vi "stream_only_production.vi"() -> ()   [LabVIEW 2025, in "LabJackEKG.lvlib"]
uses:
  LabJackEKG.lvlib
  StreamProducerLoopData.ctl
panel:
  out "Numeric":i32
  out "Direction":i64
  out "error out 2":errorcluster
  out "FLOW":T1(graph)={"Flow [L/min]"=nan, "Flow [L/min]"=nan, "Flow [L/min]"=nan}
  out "stop":bool
  in  "RMS Sampling Window [s]":dbl
  in  "TC Sampling Window [s]":dbl=0.25
  in  "error in (no error)":errorcluster
  in  "TC Offset [V]":dbl[](array[numeric])=[0.0, 0.0]
  in  "TC Scale":dbl[](array[numeric])=[1.0, 1.0]
  in  "Flow L/pulse":dbl[](array[numeric])=[1.0, 1.0, 1.0]
  in  "Flow Min. Sampling Window [s]":dbl
  in  "Flow Max. Samping Window [s]":dbl
  out "TC [degC]":dbl[](array[numeric])
  out "RMS [V]":dbl[](array[numeric])=[nan, nan, nan, nan, nan, nan]
  in  "Drum Max. Samping Window [s]":dbl=1.0
  in  "Drum Min. Sampling Window [s]":dbl=0.25
  in  "Sampling Frequency [Hz]":dbl=250.0
  in  "ms":u32=100
  out "Waveform Chart":dbl(graph)=nan
  in  "Drum Reflectors":i64=4
  out "error out":errorcluster={"status"=TRUE, "code"=8607, "source"="LJM_eStreamStart.vi"}
  in  "stop":bool
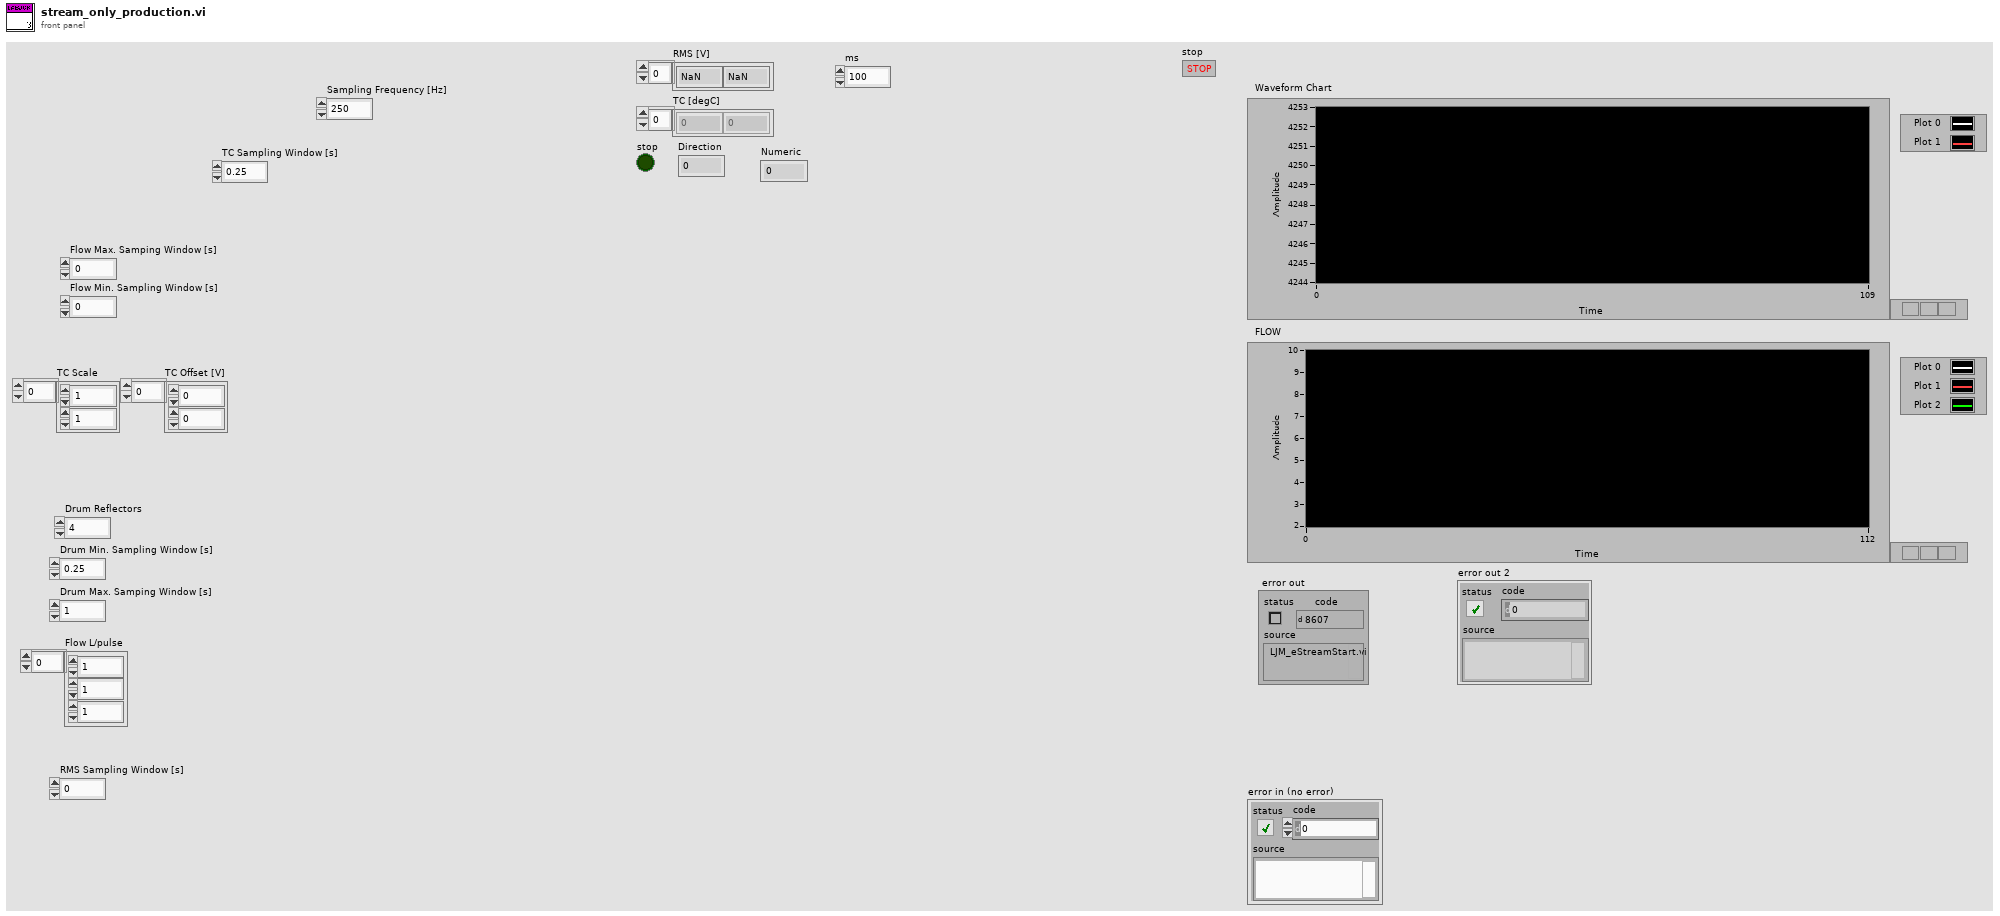
[diagram p1: front panel]
types:
  T1 = cluster{"Flow [L/min]":dbl, "Flow [L/min]":dbl, "Flow [L/min]":dbl}
  T2 = typedef "StreamProducerLoopData.ctl" = cluster{"Count":i64, "Time":i64, "Initialized":bool}
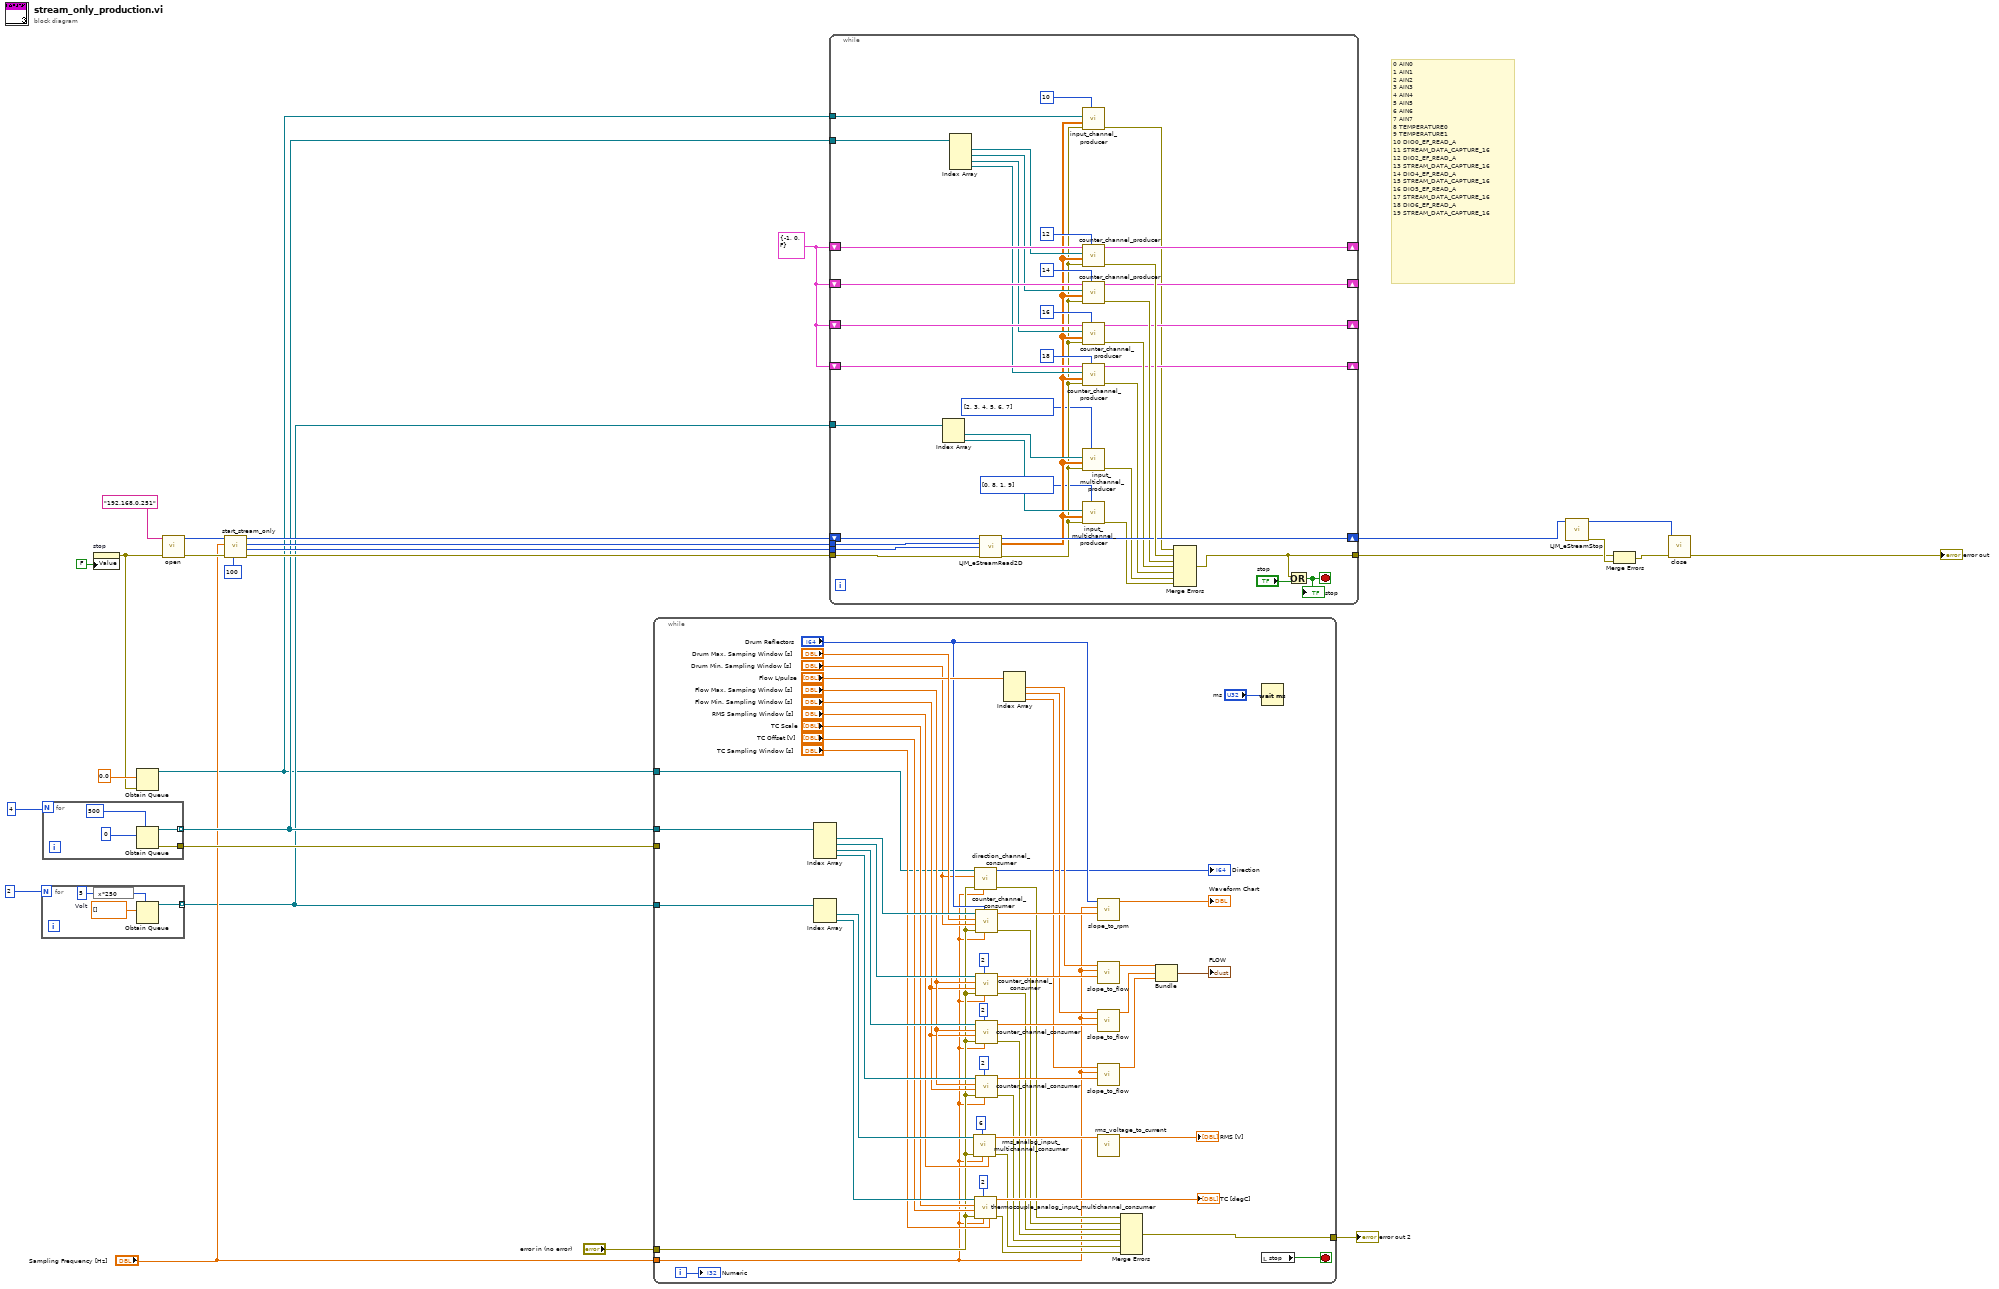
[diagram p0: block diagram]
diagram:
  w5 = T2 {"Count"=-1, "Time"=0, "Initialized"=FALSE} ("output cluster")
  # "0 AIN0\n1 AIN1\n2 AIN2\n3 AIN3\n4 AIN4\n5 AIN5\n6 AIN6\n7 AIN7\n8 TEMPERATURE0\n9 TEMPERATURE1\n10 DIO0_EF_READ_A\n11 STREAM_DATA_CAPTURE_16\n12 DIO2_EF_READ_A\n13 STREAM_DATA_CAPTURE_16\n14 DIO4_EF_READ_A\n15 STREAM_DATA_CAPTURE_16\n16 DIO5_EF_READ_A\n17 STREAM_DATA_CAPTURE_16\n18 DIO6_EF_READ_A\n19 STREAM_DATA_CAPTURE_16"
  n1 = for {
    N: 2 -> [_]
    tunnel: [w30] -> w8 mode=indexing
    w31 = dbl[] []  # Volt
    n2 = expression code="x*250"(5 ("max queue size (-1, unlimited)")) -> (w28:i32)
    n3 = Obtain Queue(max queue size (-1, unlimited)=w28, element data type=w31) -> (queue out=w30:refnum<queue>)  [unwired: 3 in, 2 out]
  }
  n4 = for {
    N: 4 -> [_]
    tunnel: [w35] -> w18
    tunnel: [w33] -> w17 mode=indexing
    n5 = Obtain Queue(max queue size (-1, unlimited)=500, element data type=i64 0) -> (queue out=w33:refnum<queue>, error out=w35:errorcluster)  [unwired: 3 in, 1 out]
  }
  n6 = property on="stop" class="Bool (strict)"("Value"=FALSE ("stop")) -> (error out=w1:errorcluster)  [unwired: 2 in, 1 out]
  n7 = Obtain Queue(element data type=0.0, error in (no error)=w1) -> (queue out=w3:refnum<queue>)  [unwired: 3 in, 2 out]
  n8 = call "open.vi"("error in"=w1, "IP Address (LJM_idANY )"="192.168.0.251") -> ("error out"=w27:errorcluster, "Handle"=w26:i32)  [unwired: 7 in, 1 out]
  n9 = call "start_stream_only.vi"("Period [ms]"=100, "error in (no error)"=w27, "Scan Rate (Hz)"="Sampling Frequency [Hz]", "Handle In"=w26) -> ("error out"=w25:errorcluster, "NumReadAddresses"=w22:i32, "ScansPerRead Out"=w23:i32, "Handle Out"=w24:i32)  [unwired: 4 in]
  n10 = while {
    tunnel: w17 -> [w83]
    tunnel: w18 -> [_]
    tunnel: "Sampling Frequency [Hz]" -> [w37]
    tunnel: w8 -> [w72]
    tunnel: "error in (no error)" -> [w40]
    tunnel: [w43] -> w6
    tunnel: w3 -> [w42]
    i -> [w36]
    stop <- w54 stop-if-true
    n11 = Index Array(array=w83) -> (element #1=w82:refnum<queue>, element #2=w81:refnum<queue>, element #3=w80:refnum<queue>, element #4=w79:refnum<queue>)  [unwired: 4 in]
    n12 = Index Array(array=w72) -> (element #1=w70:refnum<queue>, element #2=w71:refnum<queue>)  [unwired: 2 in]
    n13 = call "rms_analog_input_multichannel_consumer.vi"("Sampling Window [s]"="RMS Sampling Window [s]", "Sampling Frequency [Hz]"=w37, "Number of Channels"=6, "error in (no error)"=w40, "queue out"=w70) -> ("error out"=w48:errorcluster, "RMS [V]"=w69:dbl[])  [unwired: 5 in]
    n14 = call "direction_channel_consumer.vi"("Sampling Frequency [Hz]"=w37, "error in (no error)"=w40, "Sampling Offset [s]"="Drum Min. Sampling Window [s]", "Q"=w42) -> ("error out"=w39:errorcluster, "Direction"=→"Direction":i64)  [unwired: 6 in]
    n15 = call "thermocouple_analog_input_multichannel_consumer.vi"("Sampling Window [s]"="TC Sampling Window [s]", "Sampling Frequency [Hz]"=w37, "Number of Channels"=2, "error in (no error)"=w40, "Offset"="TC Offset [V]", "Scale"="TC Scale", "queue out"=w71) -> ("error out"=w49:errorcluster, "TC [degC]"=→"TC [degC]":dbl[])  [unwired: 1 in, 2 out]
    n16 = call "counter_channel_consumer.vi"("Sampling Frequency [Hz]"=w37, "Sample Group Size"="Drum Reflectors", "error in (no error)"=w40, "Min. Sampling Window [s]"="Drum Min. Sampling Window [s]", "Max. Samping Window [s]"="Drum Max. Samping Window [s]", "Queue in"=w82) -> ("error out"=w44:errorcluster, "slope"=w87:dbl)  [unwired: 1 in, 3 out]
    n17 = call "counter_channel_consumer.vi"("Sampling Frequency [Hz]"=w37, "Sample Group Size"=i64 2, "error in (no error)"=w40, "Min. Sampling Window [s]"="Flow Min. Sampling Window [s]", "Max. Samping Window [s]"="Flow Max. Samping Window [s]", "Queue in"=w81) -> ("error out"=w45:errorcluster, "slope"=w85:dbl)  [unwired: 1 in, 3 out]
    n18 = call "counter_channel_consumer.vi"("Sampling Frequency [Hz]"=w37, "Sample Group Size"=i64 2, "error in (no error)"=w40, "Min. Sampling Window [s]"="Flow Min. Sampling Window [s]", "Max. Samping Window [s]"="Flow Max. Samping Window [s]", "Queue in"=w80) -> ("error out"=w46:errorcluster, "slope"=w78:dbl)  [unwired: 1 in, 3 out]
    n19 = call "counter_channel_consumer.vi"("Sampling Frequency [Hz]"=w37, "Sample Group Size"=i64 2, "error in (no error)"=w40, "Min. Sampling Window [s]"="Flow Min. Sampling Window [s]", "Max. Samping Window [s]"="Flow Max. Samping Window [s]", "Queue in"=w79) -> ("error out"=w47:errorcluster, "slope"=w77:dbl)  [unwired: 1 in, 3 out]
    n20 = Index Array(array="Flow L/pulse") -> (element #1=w62:dbl, element #2=w61:dbl, element #3=w60:dbl)  [unwired: 3 in]
    n21 = call "slope_to_rpm.vi"("slope"=w87, "Sampling Frequency [Hz]"=w37, "Number of Stickers"="Drum Reflectors") -> ("RPM"=→"Waveform Chart":dbl)  [unwired: 8 in]
    n22 = call "slope_to_flow.vi"("slope"=w85, "Sampling Frequency [Hz]"=w37, "L/pulse"=w62) -> ("Flow [L/min]"=w53:dbl)  [unwired: 8 in]
    n23 = call "slope_to_flow.vi"("slope"=w78, "Sampling Frequency [Hz]"=w37, "L/pulse"=w61) -> ("Flow [L/min]"=w52:dbl)  [unwired: 8 in]
    n24 = call "slope_to_flow.vi"("slope"=w77, "Sampling Frequency [Hz]"=w37, "L/pulse"=w60) -> ("Flow [L/min]"=w51:dbl)  [unwired: 8 in]
    n25 = call "rms_voltage_to_current.vi"("RMS [V]"=w69) -> ("RMS[A]"=→"RMS [V]":dbl[])  [unwired: 10 in]
    n26 = Merge Errors(w39, w44, w45, w46, w47, w48, w49) -> (w43:errorcluster)
    n27 = Bundle("Flow [L/min]"=w53, "Flow [L/min]"=w52, "Flow [L/min]"=w51) -> (→"FLOW":T1)  [unwired: 1 in]
    n28 = Wait (ms)(milliseconds to wait="ms") -> ()  [unwired: 1 out]
    n29 = local read "stop"() -> (w54:bool)
    "Numeric" <- w36
  }
  "error out 2" <- w6
  n30 = while {
    tunnel: w25 -> [w129]
    tunnel: [w101] -> w12
    tunnel: w23 -> [w127]
    tunnel: w22 -> [w128]
    shift-right: [w122] -> w16
    shift-left: w24 -> [w126]
    tunnel: w17 -> [w106]
    shift-right: [w121] -> _
    shift-left: w5 -> [w120]
    shift-right: [w118] -> _
    shift-left: w5 -> [w117]
    shift-right: [w110] -> _
    shift-left: w5 -> [w109]
    shift-right: [w108] -> _
    shift-left: w5 -> [w107]
    tunnel: w8 -> [w99]
    tunnel: w3 -> [w91]
    stop <- w123 stop-if-true
    n31 = Index Array(array=w99) -> (element #1=w98:refnum<queue>, element #2=w97:refnum<queue>)  [unwired: 2 in]
    n32 = Index Array(array=w106) -> (element #1=w105:refnum<queue>, element #2=w104:refnum<queue>, element #3=w103:refnum<queue>, element #4=w102:refnum<queue>)  [unwired: 4 in]
    n33 = call <vilib>:"LJM_eStreamRead2D.vi"("Handle In"=w126, "ScansPerRead"=w127, "NumAddresses"=w128, "error in"=w129) -> ("Handle Out"=w122:i32, "aData Out"=w94:dbl[][], "error out"=w93:errorcluster)  [unwired: 7 in, 2 out]
    n34 = call "input_channel_producer.vi"("Index"=10 ("Channel"), "error in (no error)"=w93, "aData Out"=w94, "Q"=w91) -> ("error out"=w92:errorcluster)  [unwired: 7 in]
    n35 = call "counter_channel_producer.vi"("Channel"=12 ("disabled index (col)"), "error in (no error)"=w93, "aData Out"=w94, "Queue in"=w105, "output cluster in"=w120) -> ("error out"=w124:errorcluster, "output cluster out"=w121:T2)  [unwired: 5 in]
    n36 = call "counter_channel_producer.vi"("Channel"=14 ("disabled index"), "error in (no error)"=w93, "aData Out"=w94, "Queue in"=w104, "output cluster in"=w117) -> ("error out"=w115:errorcluster, "output cluster out"=w118:T2)  [unwired: 5 in]
    n37 = call "counter_channel_producer.vi"("Channel"=16 ("disabled index"), "error in (no error)"=w93, "aData Out"=w94, "Queue in"=w103, "output cluster in"=w109) -> ("error out"=w111:errorcluster, "output cluster out"=w110:T2)  [unwired: 5 in]
    n38 = call "counter_channel_producer.vi"("Channel"=18 ("disabled index"), "error in (no error)"=w93, "aData Out"=w94, "Queue in"=w102, "output cluster in"=w107) -> ("error out"=w112:errorcluster, "output cluster out"=w108:T2)  [unwired: 5 in]
    n39 = call "input_multichannel_producer.vi"("Indices"=i32[] [2, 3, 4, 5, 6, 7], "error in (no error)"=w93, "aData Out"=w94, "Q"=w98) -> ("error out"=w100:errorcluster)  [unwired: 7 in]
    n40 = call "input_multichannel_producer.vi"("Indices"=i32[] [0, 8, 1, 9], "error in (no error)"=w93, "aData Out"=w94, "Q"=w97) -> ("error out"=w96:errorcluster)  [unwired: 7 in]
    n41 = Merge Errors(w92, w124, w115, w111, w112, w100, w96) -> (w101:errorcluster)
    n42 = Or(x=w101, y="stop") -> (x .or. y?=w123:bool)
    "stop" <- w123
  }
  n43 = call <vilib>:"LJM_eStreamStop.vi"("Handle In"=w16) -> ("Handle Out"=w15:i32, "error out"=w13:errorcluster)  [unwired: 13 in]
  n44 = Merge Errors(w12, w13) -> (w14:errorcluster)
  n45 = call "close.vi"("error in"=w14, "Handle"=w15) -> ("error out"=→"error out":errorcluster)  [unwired: 9 in]
